vi "TB3000_frequency_query.vi"(7 "unit":enum16{"Hz", "kHz", "MHz"}(ring), 11 "VISA resource name in":refnum<visa-resource-name>) -> (2 "frequency":dbl, 3 "VISA resource name out":refnum<visa-resource-name>)   [LabVIEW 2021]
panel:
  out "Error Out":errorcluster
  in  "Error In":errorcluster
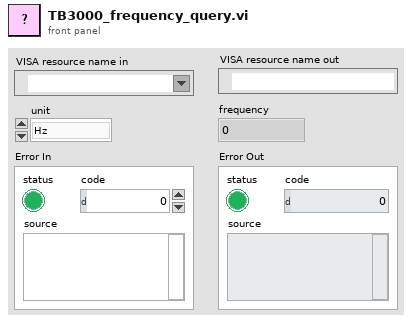
[diagram p1: front panel]
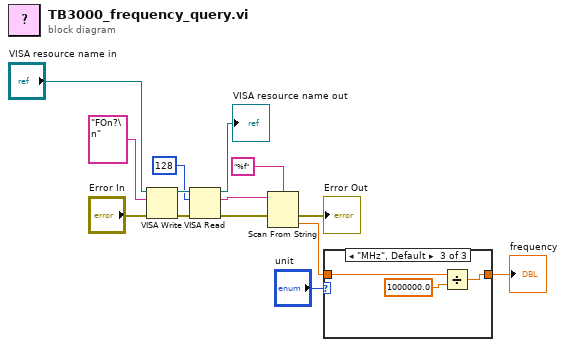
[diagram p0: block diagram]
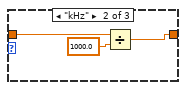
[diagram p3: hidden frame]
diagram:
  n1 = VISA Write(VISA resource name="VISA resource name in", write buffer="FOn?\n", error in (no error)="Error In") -> (VISA resource name out=w13:refnum<visa-resource-name>, error out=w12:errorcluster)  [unwired: 1 out]
  n2 = VISA Read(VISA resource name=w13, byte count=u32 128, error in (no error)=w12) -> (VISA resource name out=→"VISA resource name out":refnum<visa-resource-name>, read buffer=w7:string, error out=w6:errorcluster)  [unwired: 1 out]
  n3 = Scan From String(format string="%f", input string=w7, error in=w6) -> (error out=→"Error Out":errorcluster, output 1=w5:dbl)  [unwired: 2 in, 2 out]
  n4 = case shown="\"MHz\", Default" "unit" {
    tunnel: w5 -> [w15 w18 w20]
    tunnel: [w15 w17 w19] -> w4
    frame "Hz" {
    }
    frame "kHz" {
      n5 = Divide(x=w18, y=1000.0) -> (x/y=w17:dbl)
    }
    frame "MHz", Default {
      n6 = Divide(x=w20, y=1000000.0) -> (x/y=w19:dbl)
    }
  }
  "frequency" <- w4
